vi "TCP Write Alive.vi"() -> ()   [LabVIEW 2011]
uses:
  <vilib>/Utility/tcp.llb/UDP Multicast Read-Only Open.vi
panel:
  in  "remote port or service name 2":u16=6341
  in  "address 2":string="localhost"
  in  "Name 2":string="MyName2>>"
  in  "OK":bool
  in  "MultiCast Address":string="234.5.6.7"
  out "Stopped":bool
  in  "MultiCast Port":u16=58432
  out "NaN/Path/Refnum? 2":bool
  out "concatenated string":string
  out "NaN/Path/Refnum?":bool
  in  "stop":bool
  in  "Name":string="MyName2>>"
  in  "Wait for Stop?":bool
  out "data out":string
  in  "remote port or service name":u16=6341
  in  "address":string="localhost"
  in  "timeout ms (25000)":i32
  out "connection ID out":refnum<k5>
  out "error out":errorcluster
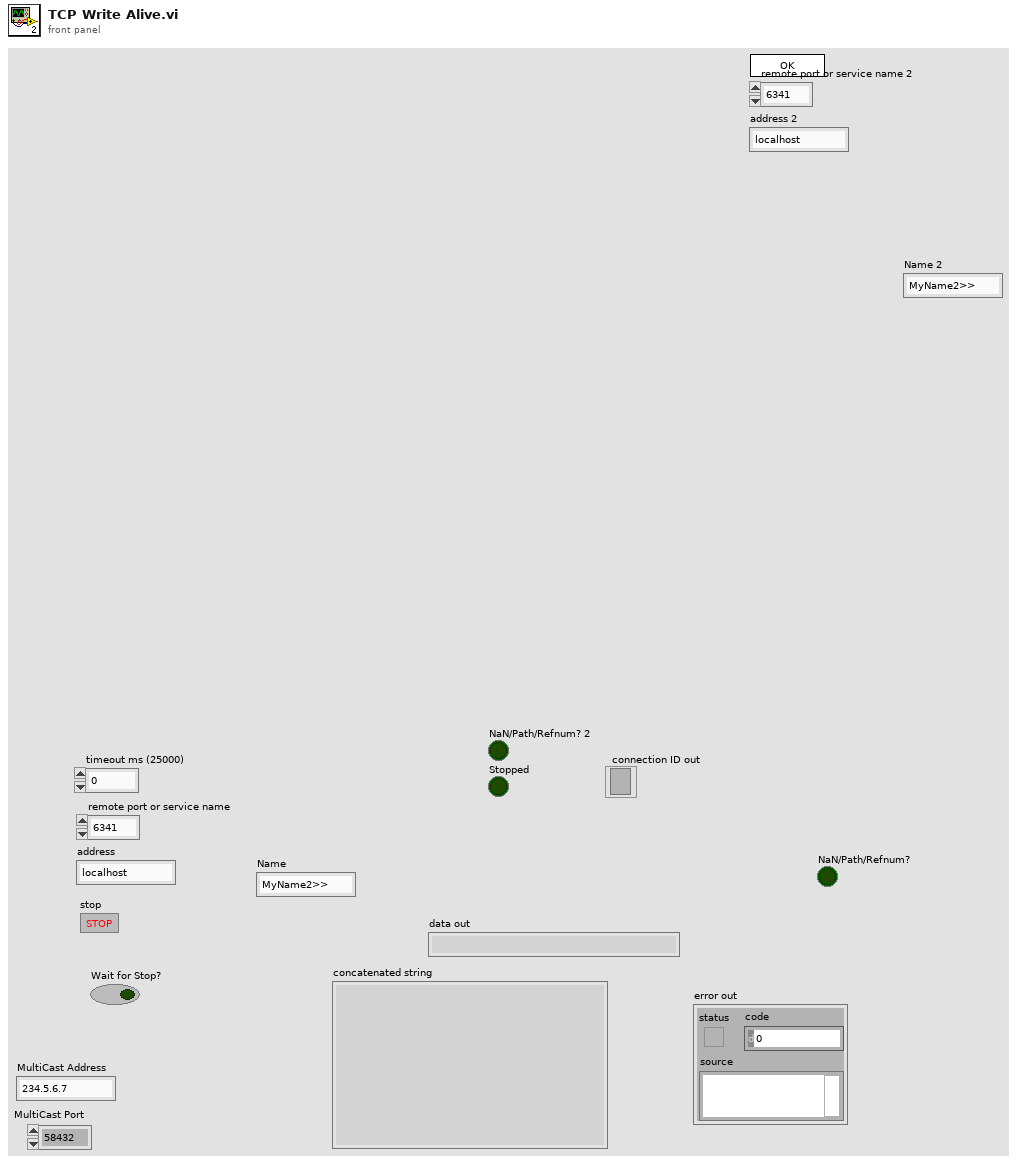
[diagram p1: front panel]
types:
  T1 = enum32{"invalid app kind", "Development System", "Run Time System", "Student Edition", "Embedded LabVIEW", "Evaluation", "Custom"}
  T2 = enum32{"Invalid", "Standard", "Closed", "Hidden", "Minimized", "Maximized"}
  T3 = cluster{"Core":cluster{"Current VI Reference":refnum<vi>, "Close Panel on Exit?":bool}, "Your Boolean data":bool, "Alive String":string, "connection ID":refnum<k5>, "Address":string, "remote port or service name 2":u16, "Stop String":string}
  T4 = cluster{"Current VI Reference":refnum<vi>, "Close Panel on Exit?":bool}
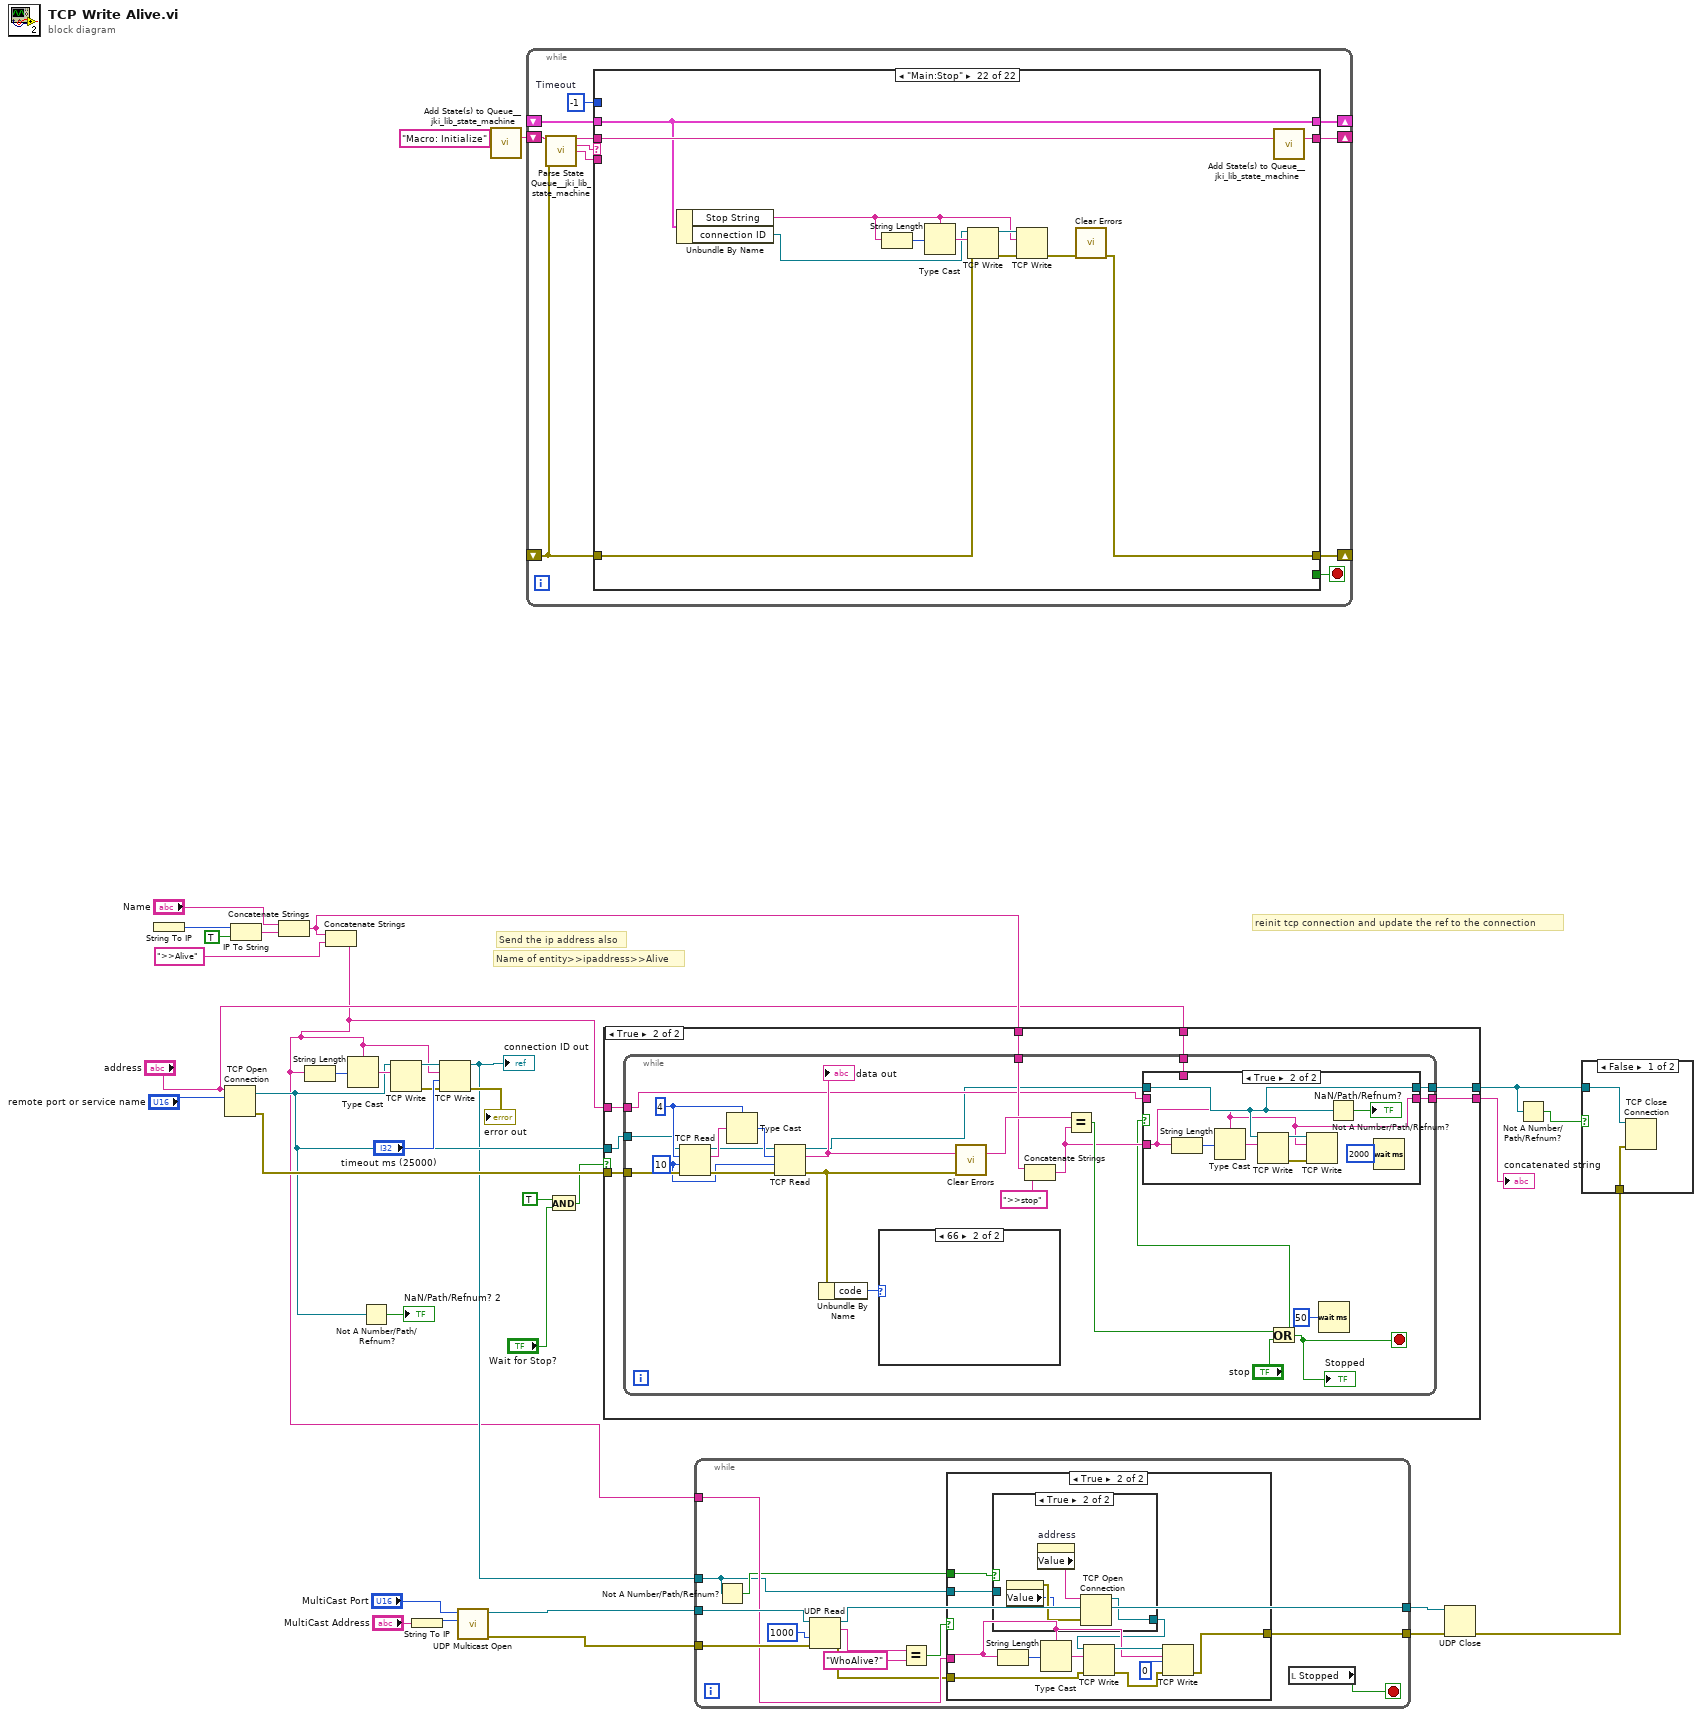
[diagram p0: block diagram]
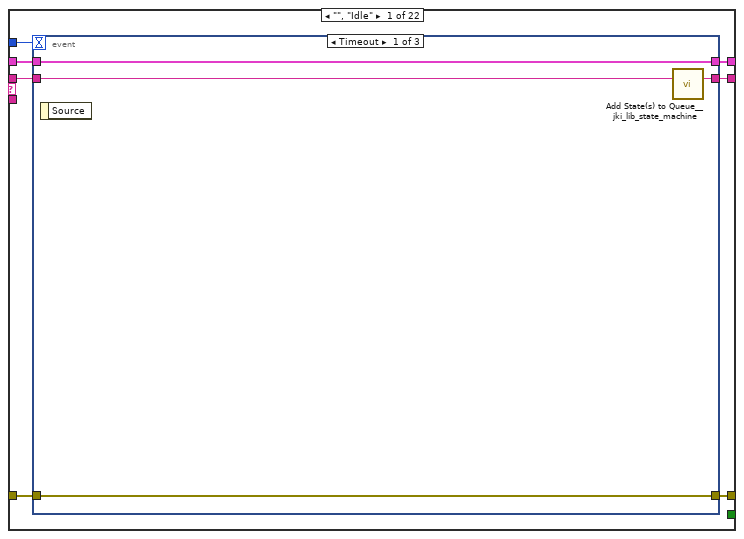
[diagram p2: hidden frame]
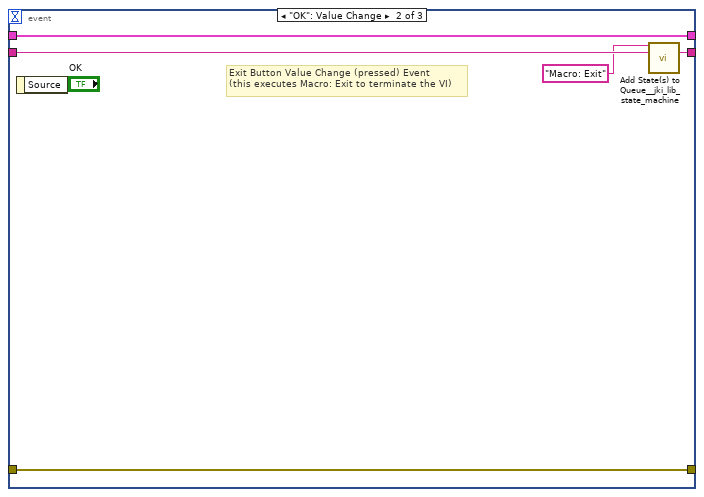
[diagram p3: hidden frame]
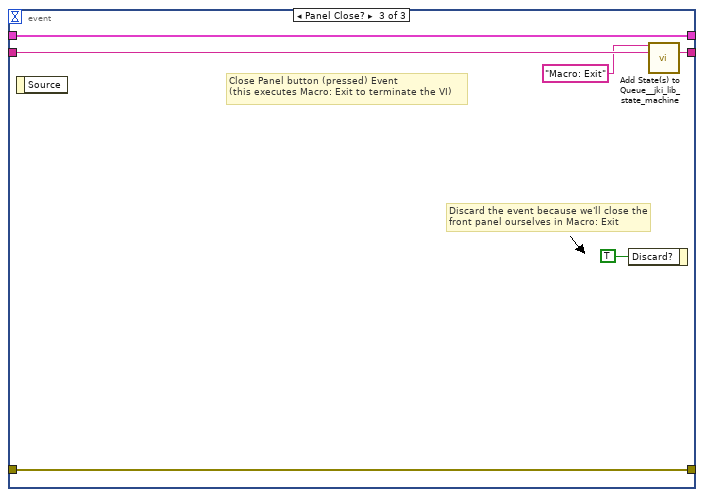
[diagram p4: hidden frame]
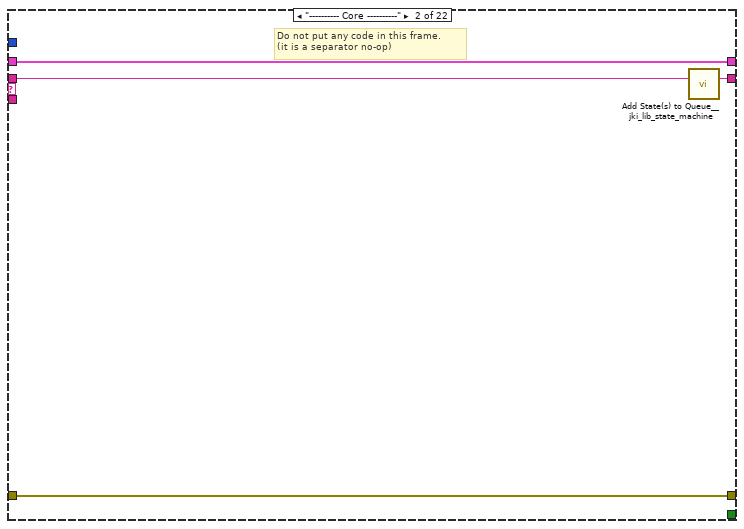
[diagram p5: hidden frame]
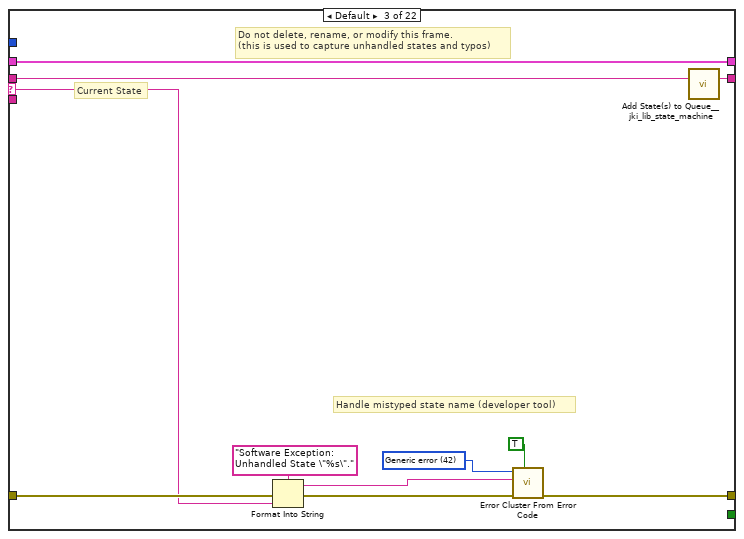
[diagram p6: hidden frame]
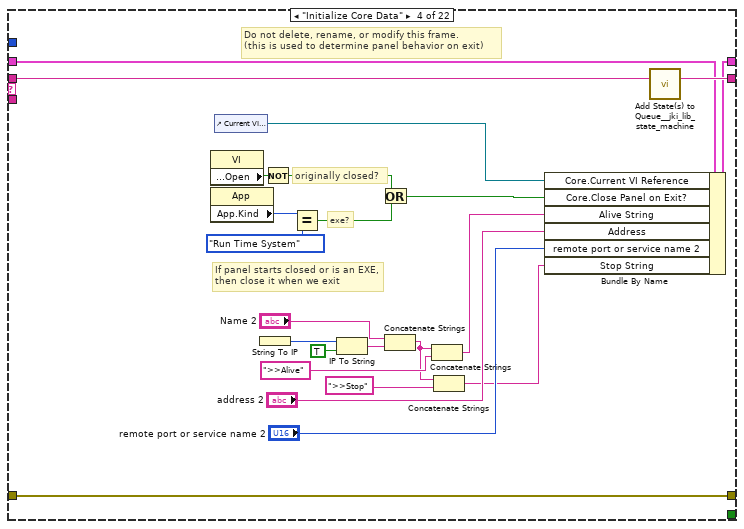
[diagram p7: hidden frame]
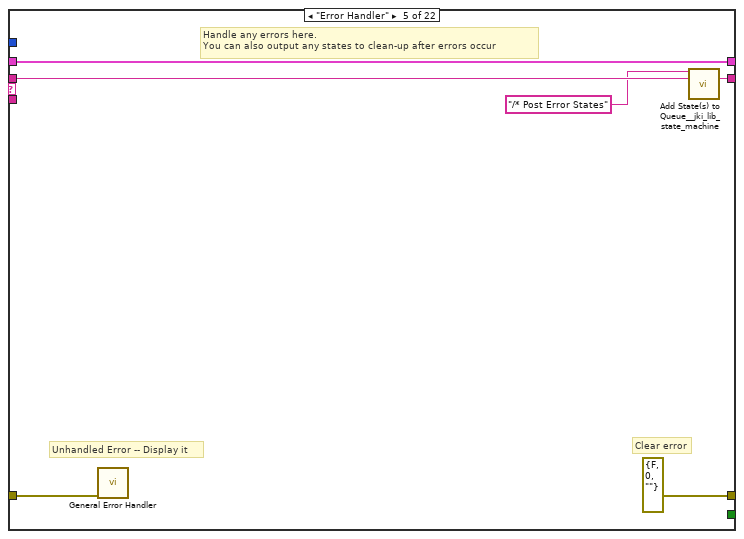
[diagram p8: hidden frame]
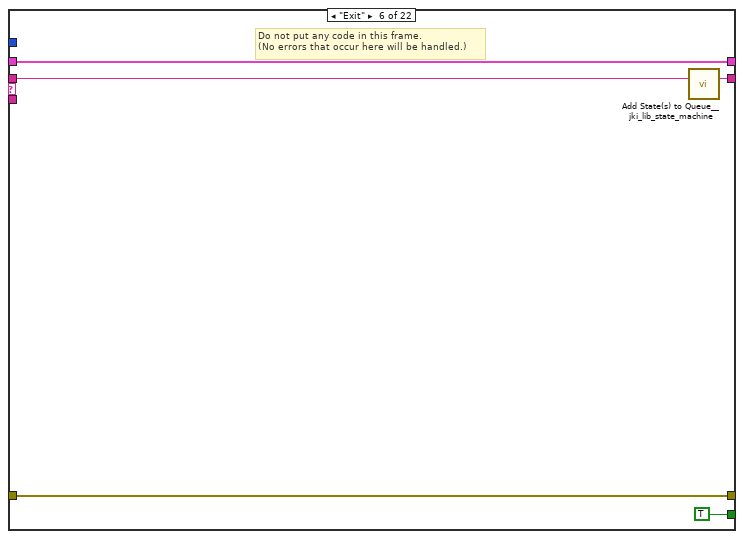
[diagram p9: hidden frame]
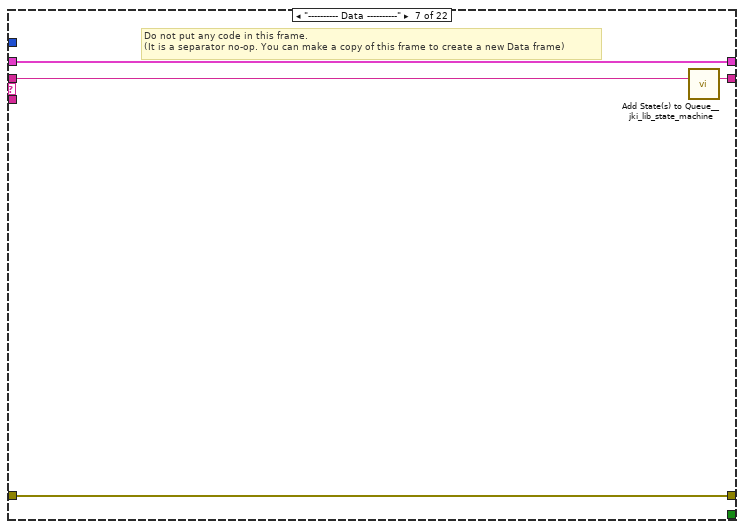
[diagram p10: hidden frame]
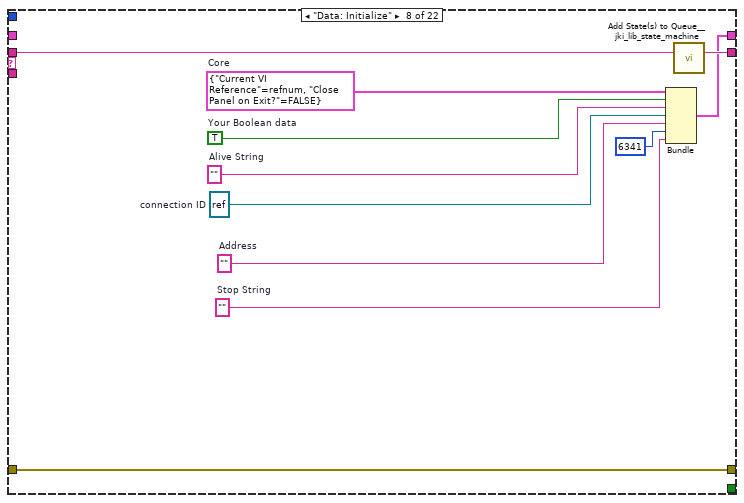
[diagram p11: hidden frame]
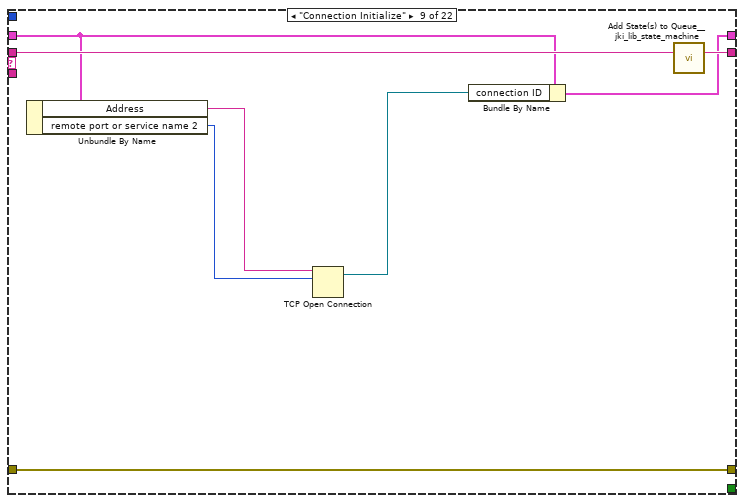
[diagram p12: hidden frame]
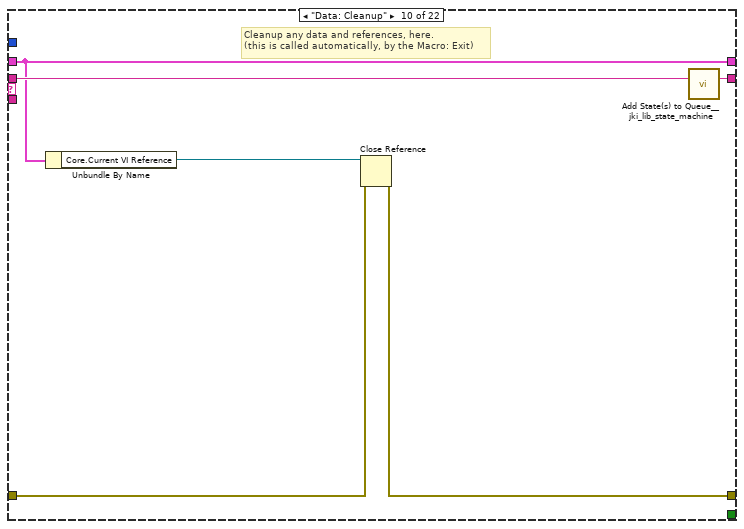
[diagram p13: hidden frame]
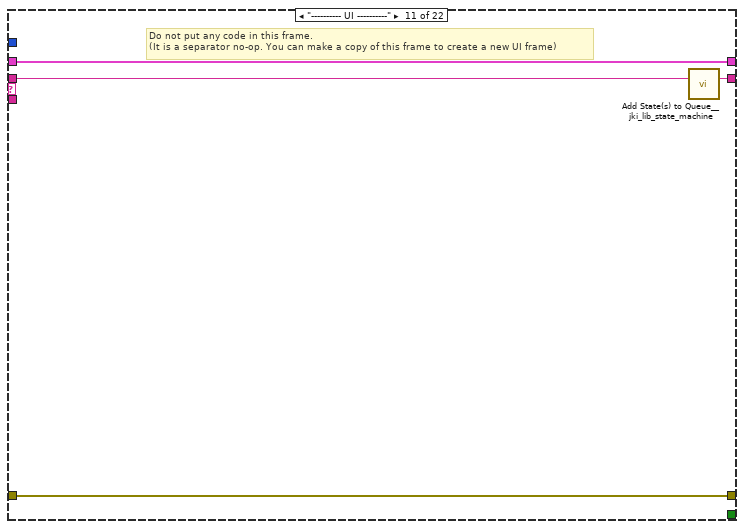
[diagram p14: hidden frame]
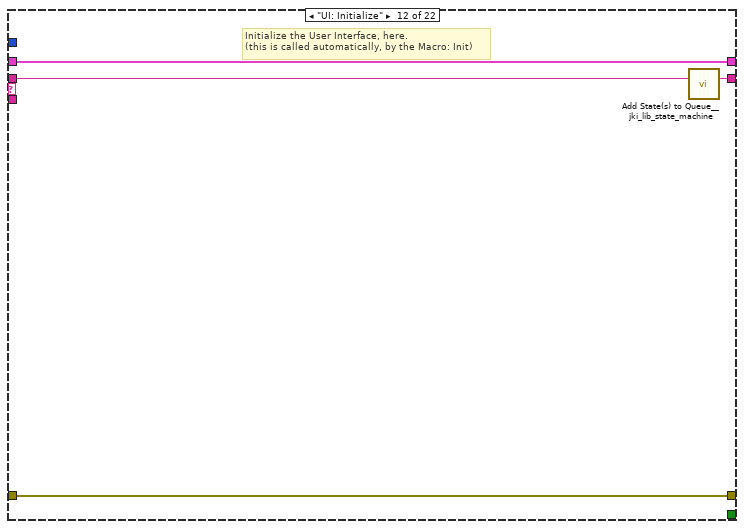
[diagram p15: hidden frame]
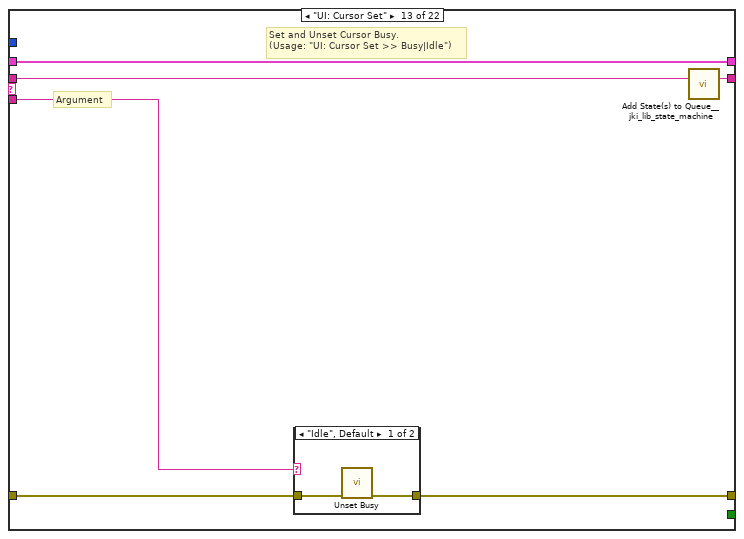
[diagram p16: hidden frame]
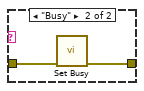
[diagram p17: hidden frame]
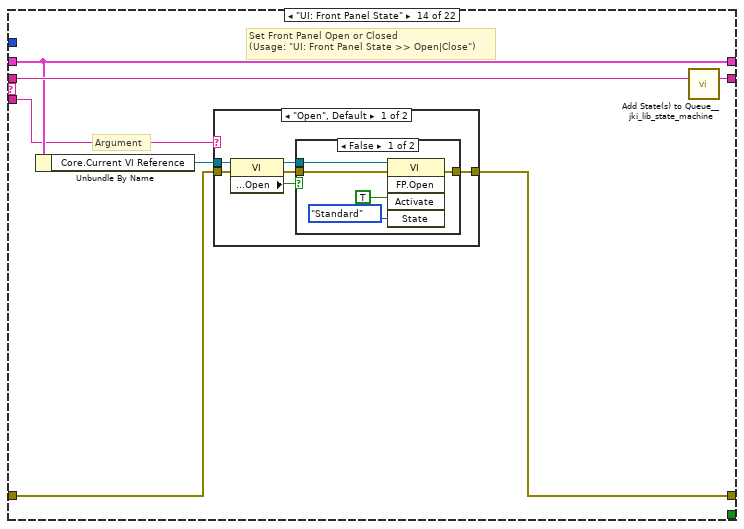
[diagram p18: hidden frame]
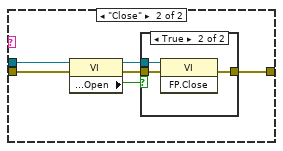
[diagram p20: hidden frame]
diagram:
  # "reinit tcp connection and update the ref to the connection"
  # "Send the ip address also"
  # "Name of entity>>ipaddress>>Alive"
  n1 = String To IP() -> (0:w24:u32)  [unwired: 1 in]
  n2 = TCP Open Connection(address="address", remote port or service name="remote port or service name") -> (connection ID=w15:refnum<k5>, error out=w29:errorcluster)  [unwired: 3 in]
  n3 = IP To String(1:TRUE ("dot notation? (F)"), 2:w24) -> (0:w22:string)
  n4 = Concatenate Strings("Name", w22) -> (w20:string)
  n5 = Concatenate Strings(w20, ">>Alive" ("string")) -> (w8:string)
  n6 = String Length(string=w8) -> (length=w31:i32)
  n7 = Type Cast(type=w8, x=w31) -> (*(type *) &x=w30:string)
  n8 = Not A Number/Path/Refnum?(number/path/refnum=w15) -> (NaN/Path/Refnum?=→"NaN/Path/Refnum? 2":bool)
  n9 = TCP Write(connection ID=w15, data in=w30) -> (connection ID out=w33:refnum<k5>, error out=w32:errorcluster)  [unwired: 2 in, 1 out]
  n10 = String To IP(1:"MultiCast Address") -> (0:w4:u32)
  n11 = TCP Write(connection ID=w33, data in=w8, error in (no error)=w32, 9:"timeout ms (25000)") -> (connection ID out=w9:refnum<k5>, error out=→"error out":errorcluster)  [unwired: 1 out]
  "connection ID out" <- w9
  n12 = call-poly <vilib>:"UDP Multicast Open.vi"("multicast addr"=w4, "port"="MultiCast Port") -> ("error out"=w11:errorcluster, "connection ID"=w10:refnum<k16>)  [unwired: 7 in, 1 out]
  n13 = call <vilib>:"Add State(s) to Queue__jki_lib_state_machine.vi"("State(s) in (\"\")"="Macro: Initialize") -> ("States Out"=w2:string)  [unwired: 14 in]
  n14 = while {
    shift-right: [w39] -> _
    shift-left: _ -> [w38]
    shift-right: [w42] -> _
    shift-left: _ -> [w36]
    shift-right: [w41] -> _
    shift-left: w2 -> [w43]
    stop <- w40 stop-if-true
    w37 = -1  # Timeout
    n15 = call <vilib>:"Parse State Queue__jki_lib_state_machine.vi"("State Queue"=w43, "Error In (no error)"=w36) -> ("Remaining States"=w45:string, "Current State"=w46:string, "Arguments"=w44:string)  [unwired: 11 in]
    n16 = case shown="\"Main:Stop\"" w46 {
      selector: w46 -> [_ _ w73 _ _ _ _ _ _ _ _ _ _ _ _ _ _ _ _ _ _ _]
      tunnel: w45 -> [w53 w72 w77 w106 w112 w117 w121 w132 w140 w146 w150 w154 w160 w171 w197 w202 w212 w216 w225 w242 w265 w277]
      tunnel: w44 -> [_ _ _ _ _ _ _ _ _ _ _ _ w155 w165 _ _ _ _ _ _ _ _]
      tunnel: w38 -> [w51 w69 w75 w97 w109 w115 w118 _ w135 w141 w147 w152 w158 w167 w194 w199 w209 w213 w219 w233 w259 w271]
      tunnel: [w50 w70 w79 w103 errorcluster {"status"=FALSE, "code"=0, "source"=""} ("error out") w114 w119 w129 w138 w142 w148 w151 w156 w168 w195 w200 w210 w214 w223 w227 w254 w266] -> w42
      tunnel: w36 -> [w49 w70 w78 w103 w108 w114 w119 w129 w138 w143 w148 w151 w157 w169 w195 w200 w210 w214 w223 w228 w256 w268]
      tunnel: [w52 w71 w76 w105 w111 w116 w120 w131 w139 w145 w149 w153 w159 w170 w196 w201 w211 w215 w224 w241 w264 w276] -> w41
      tunnel: [_ _ _ _ _ TRUE _ _ _ _ _ _ _ _ _ _ _ _ _ _ _ _] -> w40
      tunnel: [w48 w69 w75 w104 w109 w115 w118 w130 w137 w141 w147 w152 w158 w167 w194 w199 w209 w213 w218 w233 w259 w271] -> w39
      tunnel: w37 -> [w47 _ _ _ _ _ _ _ _ _ _ _ _ _ _ _ _ _ _ _ _ _]
      frame "", "Idle" {
        n17 = event shown="[0] Timeout" {
          selector: _ -> [_ _ _]
          dyn-events: _ -> [_ _ _]
          timeout: w47 -> [_ _ _]
          tunnel: w53 -> [w57 w62 w68]
          tunnel: [w56 w61 w67] -> w52
          tunnel: w51 -> [w54 w59 w65]
          tunnel: [w55 w60 w66] -> w50
          tunnel: w49 -> [w55 w60 w66]
          tunnel: [w54 w59 w65] -> w48
          event Timeout {
            n18 = event-data() -> ()  [unwired: 1 in, 1 out]
            n19 = call <vilib>:"Add State(s) to Queue__jki_lib_state_machine.vi"("State(s) in (\"\")"=w57) -> ("States Out"=w56:string)  [unwired: 14 in]
          }
          event "OK": Value Change {
            # "Exit Button Value Change (pressed) Event\n(this executes Macro: Exit to terminate the VI)"
            n20 = event-data() -> ()  [unwired: 1 in, 1 out]
            n21 = call <vilib>:"Add State(s) to Queue__jki_lib_state_machine.vi"("State(s) in Front (\"\")"="Macro: Exit", "State(s) in (\"\")"=w62) -> ("States Out"=w61:string)  [unwired: 13 in]
          }
          event Panel Close? {
            # "Discard the event because we'll close the front panel ourselves in Macro: Exit"
            # "Close Panel button (pressed) Event\n(this executes Macro: Exit to terminate the VI)"
            n22 = event-data() -> ()  [unwired: 1 in, 1 out]
            n23 = event-data("Discard?"=TRUE) -> ()  [unwired: 1 in, 1 out]
            n24 = call <vilib>:"Add State(s) to Queue__jki_lib_state_machine.vi"("State(s) in Front (\"\")"="Macro: Exit", "State(s) in (\"\")"=w68) -> ("States Out"=w67:string)  [unwired: 13 in]
          }
        }
      }
      frame "---------- Core ----------" {
        # "Do not put any code in this frame.\n(it is a separator no-op)"
        n25 = call <vilib>:"Add State(s) to Queue__jki_lib_state_machine.vi"("State(s) in (\"\")"=w72) -> ("States Out"=w71:string)  [unwired: 14 in]
      }
      frame Default {
        w82 = 42 items=["No error", "Argument error", "Memory is full", "Out of zone", "End of file", "File already open", "Generic file I/O error", "File not found", "File permission error", "Disk is full", "Duplicate path", "Too many files open", "System feature not enabled", "Resource file not found", "Cannot add resource", "Resource not found", "Image not found", "Image memory error", "Pen does not exist", "Config type invalid", "Config token not found", "Config parse error", "Config memory error", "Bad external code format", "Bad external code offset", "External code not present", "Null window", "Destroy window error", "Null menu", "Print aborted", "Bad print record", "Print driver error", "Windows error during printing", "Memory error during printing", "Print dialog error", "Generic print error", "Invalid device refnum", "Device not found", "Device parameter error", "Device unit error", "Cannot open device", "Device call aborted", "Generic error", "Cancelled by user", "Object ID too low", "Object ID too high", "Object not in heap", "Unknown heap", "Unknown object (invalid DefProc)", "Unknown object (DefProc not in table)", "Message out of range", "Invalid (null) method", "Unknown message", "Manager call not supported", "Bad address", "Network operation in progress", "Network operation timed out", "Connection is busy", "Network attribute not supported", "Network error", "Address in use", "System out of memory", "Connection aborted", "Connection refused", "Not connected", "Already connected", "Connection closed", "Initialization error (interapplication manager)", "Bad occurrence", "Wait on unbound occurrence handler", "Occurrence queue overflow", "Datalog type conflict", "Unused", "Unrecognized type (interapplication manager)", "Memory corrupt", "Failed to make temporary DLL", "Old CIN version", "Drag socket not found", "Failed to load drop-object", "Failed to register OLE object", "Failed to release OLE object", "Format specifier type mismatch", "Unknown format specifier", "Too few format specifiers", "Too many format specifiers", "Scan failed", "Newer CIN version", "Error converting to variant", "Runtime menu error", "Password tampered", "Variant attribute not found", "Incompatible variant data type", "Event data is not available", "Event Store is not present", "Occurrence is not found", "Event Queue is not created", "Event info is not available", "Refnum passed is NULL", "Error retrieving Class GUID", "Error retrieving CoClass GUID", "Error retrieving TypeLib GUID.", "Bad built application magic bytes.", "Specific driver is different from the specific driver associated with the Logical Name.", "There is no session opened to the class driver.", "Max Error", "MAX - Error with config objects", "MAX - Error loading configuration", "MAX - Group not supported"]
        # "Current State"
        # "Do not delete, rename, or modify this frame.\n(this is used to capture unhandled states and typos)"
        # "Handle mistyped state name (developer tool)"
        n26 = Format Into String(format string="Software Exception: Unhandled State \"%s\"." ("message"), error in=w78, w73) -> (resulting string=w81:string, error out=w80:errorcluster)  [unwired: 1 in]
        n27 = call <vilib>:"Error Cluster From Error Code.vi"("show call chain? (False)"=TRUE, "error in (no error)"=w80, "error message (\"\")"=w81, "error code (0)"=w82) -> ("error out"=w79:errorcluster)  [unwired: 5 in]
        n28 = call <vilib>:"Add State(s) to Queue__jki_lib_state_machine.vi"("State(s) in (\"\")"=w77) -> ("States Out"=w76:string)  [unwired: 14 in]
      }
      frame "Initialize Core Data" {
        # "Do not delete, rename, or modify this frame.\n(this is used to determine panel behavior on exit)"
        # "originally closed?"
        # "exe?"
        # "If panel starts closed or is an EXE, then close it when we exit"
        n29 = property class="VI"() -> ("Front Panel.Open"=w102:bool)  [unwired: 2 in, 2 out]
        n30 = property class="App"() -> ("App.Kind"=w101:T1)  [unwired: 2 in, 2 out]
        n31 = control-ref of="Current VI Reference"() -> (w95:refnum<vi>)
        n32 = String To IP() -> (0:w91:u32)  [unwired: 1 in]
        n33 = Not(x=w102) -> (.not. x?=w99:bool)
        n34 = Equal?(x=w101, y=T1."Run Time System" ("Application:Kind")) -> (x = y?=w98:bool)
        n35 = IP To String(1:TRUE ("dot notation? (F)"), 2:w91) -> (0:w93:string)
        n36 = Or(x=w99, y=w98) -> (x .or. y?=w96:bool)
        n37 = Concatenate Strings("Name 2", w93) -> (w86:string)
        n38 = Concatenate Strings(w86, ">>Alive" ("string")) -> (w87:string)
        n39 = Concatenate Strings(w86, ">>Stop" ("string")) -> (w84:string)
        n40 = Bundle By Name(cluster=w97, "Core.Current VI Reference"=w95, "Core.Close Panel on Exit?"=w96, "Alive String"=w87, "Address"="address 2", "remote port or service name 2"="remote port or service name 2", "Stop String"=w84) -> (w104:T3)
        n41 = call <vilib>:"Add State(s) to Queue__jki_lib_state_machine.vi"("State(s) in (\"\")"=w106) -> ("States Out"=w105:string)  [unwired: 14 in]
      }
      frame "Error Handler" {
        # "Unhandled Error -- Display it"
        # "Handle any errors here.\nYou can also output any states to clean-up after errors occur"
        # "Clear error"
        n42 = call <vilib>:"General Error Handler.vi"("error in (no error)"=w108) -> ()  [unwired: 10 in, 5 out]
        n43 = call <vilib>:"Add State(s) to Queue__jki_lib_state_machine.vi"("State(s) in Front (\"\")"="/* Post Error States", "State(s) in (\"\")"=w112) -> ("States Out"=w111:string)  [unwired: 13 in]
      }
      frame "Exit" {
        # "Do not put any code in this frame.\n(No errors that occur here will be handled.)"
        n44 = call <vilib>:"Add State(s) to Queue__jki_lib_state_machine.vi"("State(s) in (\"\")"=w117) -> ("States Out"=w116:string)  [unwired: 14 in]
      }
      frame "---------- Data ----------" {
        # "Do not put any code in this frame.\n(It is a separator no-op. You can make a copy of this frame to create a new Data frame)"
        n45 = call <vilib>:"Add State(s) to Queue__jki_lib_state_machine.vi"("State(s) in (\"\")"=w121) -> ("States Out"=w120:string)  [unwired: 14 in]
      }
      frame "Data: Initialize" {
        w122 = ""  # Stop String
        w124 = ""  # Address
        w125 = refnum<k5> refnum  # connection ID
        w126 = T4 {"Current VI Reference"=refnum, "Close Panel on Exit?"=FALSE}  # Core
        w128 = TRUE  # Your Boolean data
        w127 = ""  # Alive String
        n46 = Bundle("Core"=w126, "Your Boolean data"=w128, "Alive String"=w127, "connection ID"=w125, "Address"=w124, "remote port or service name 2"=u16 6341, "Stop String"=w122) -> (w130:T3)  [unwired: 1 in]
        n47 = call <vilib>:"Add State(s) to Queue__jki_lib_state_machine.vi"("State(s) in (\"\")"=w132) -> ("States Out"=w131:string)  [unwired: 14 in]
      }
      frame "Connection Initialize" {
        n48 = Unbundle By Name(w135) -> ("Address"=w134:string, "remote port or service name 2"=w133:u16)
        n49 = TCP Open Connection(address=w134, remote port or service name=w133) -> (connection ID=w136:refnum<k5>)  [unwired: 3 in, 1 out]
        n50 = Bundle By Name(cluster=w135, "connection ID"=w136) -> (w137:T3)
        n51 = call <vilib>:"Add State(s) to Queue__jki_lib_state_machine.vi"("State(s) in (\"\")"=w140) -> ("States Out"=w139:string)  [unwired: 14 in]
      }
      frame "Data: Cleanup" {
        # "Cleanup any data and references, here.\n(this is called automatically, by the Macro: Exit)"
        n52 = Unbundle By Name(w141) -> ("Core.Current VI Reference"=w144:refnum<vi>)
        n53 = Close Reference(reference=w144, error in (no error)=w143) -> (error out=w142:errorcluster)
        n54 = call <vilib>:"Add State(s) to Queue__jki_lib_state_machine.vi"("State(s) in (\"\")"=w146) -> ("States Out"=w145:string)  [unwired: 14 in]
      }
      frame "---------- UI ----------" {
        # "Do not put any code in this frame.\n(It is a separator no-op. You can make a copy of this frame to create a new UI frame)"
        n55 = call <vilib>:"Add State(s) to Queue__jki_lib_state_machine.vi"("State(s) in (\"\")"=w150) -> ("States Out"=w149:string)  [unwired: 14 in]
      }
      frame "UI: Initialize" {
        # "Initialize the User Interface, here.\n(this is called automatically, by the Macro: Init)"
        n56 = call <vilib>:"Add State(s) to Queue__jki_lib_state_machine.vi"("State(s) in (\"\")"=w154) -> ("States Out"=w153:string)  [unwired: 14 in]
      }
      frame "UI: Cursor Set" {
        # "Argument"
        # "Set and Unset Cursor Busy.\n(Usage: \"UI: Cursor Set >> Busy|Idle\")"
        n57 = case shown="\"Idle\", Default" w155 {
          tunnel: w157 -> [w162 w164]
          tunnel: [w161 w163] -> w156
          frame "Idle", Default {
            n58 = call <vilib>:"Unset Busy.vi"("error in (no error)"=w162) -> ("error out"=w161:errorcluster)  [unwired: 10 in]
          }
          frame "Busy" {
            n59 = call <vilib>:"Set Busy.vi"("error in (no error)"=w164) -> ("error out"=w163:errorcluster)  [unwired: 9 in, 1 out]
          }
        }
        n60 = call <vilib>:"Add State(s) to Queue__jki_lib_state_machine.vi"("State(s) in (\"\")"=w160) -> ("States Out"=w159:string)  [unwired: 14 in]
      }
      frame "UI: Front Panel State" {
        # "Argument"
        # "Set Front Panel Open or Closed\n(Usage: \"UI: Front Panel State >> Open|Close\")"
        n61 = Unbundle By Name(w167) -> ("Core.Current VI Reference"=w166:refnum<vi>)
        n62 = case shown="\"Open\", Default" w165 {
          tunnel: w169 -> [w175 w188]
          tunnel: [w177 w189] -> w168
          tunnel: w166 -> [w176 w186]
          frame "Open", Default {
            n63 = property class="VI"(reference=w176, error in=w175) -> (reference out=w173:refnum<vi>, error out=w174:errorcluster, "Front Panel.Open"=w172:bool)
            n64 = case shown="False" w172 {
              tunnel: [w180 w183] -> w177
              tunnel: w174 -> [w179 w183]
              tunnel: w173 -> [w178 _]
              frame False {
                n65 = invoke class="VI" method="FP.Open"(reference=w178, error in=w179, "Activate"=TRUE, "State"=T2."Standard") -> (error out=w180:errorcluster)  [unwired: 1 in, 4 out]
              }
              frame True {
              }
            }
          }
          frame "Close" {
            n66 = property class="VI"(reference=w186, error in=w188) -> (reference out=w185:refnum<vi>, error out=w187:errorcluster, "Front Panel.Open"=w184:bool)
            n67 = case shown="True" w184 {
              tunnel: [w190 w193] -> w189
              tunnel: w187 -> [w190 w192]
              tunnel: w185 -> [_ w191]
              frame False {
              }
              frame True {
                n68 = invoke class="VI" method="FP.Close"(reference=w191, error in=w192) -> (error out=w193:errorcluster)  [unwired: 1 in, 2 out]
              }
            }
          }
        }
        n69 = call <vilib>:"Add State(s) to Queue__jki_lib_state_machine.vi"("State(s) in (\"\")"=w171) -> ("States Out"=w170:string)  [unwired: 14 in]
      }
      frame "---------- Macro ----------" {
        # "Do not put any code in this frame.\n(It is a separator no-op. You can make a copy of this frame to create a new Macro frame)"
        n70 = call <vilib>:"Add State(s) to Queue__jki_lib_state_machine.vi"("State(s) in (\"\")"=w197) -> ("States Out"=w196:string)  [unwired: 14 in]
      }
      frame "Macro: Initialize" {
        w198 = "Data: Initialize\nInitialize Core Data\nConnection Initialize\nUI: Initialize\nUI: Front Panel State >> Open"  # Data: Initialize Initialize Core Data Connection Initialize UI: Initialize UI: Front Panel State >> Open
        # "Initialization Macro\n(This is called once, when the VI starts)"
        n71 = call <vilib>:"Add State(s) to Queue__jki_lib_state_machine.vi"("State(s) in Front (\"\")"=w198, "State(s) in (\"\")"=w202) -> ("States Out"=w201:string)  [unwired: 13 in]
      }
      frame "Macro: Exit" {
        # "Exit Macro\n(This is called once, when the VI exits)"
        n72 = Unbundle By Name(w209) -> ("Core.Close Panel on Exit?"=w208:bool)
        n73 = Select(t="UI: Front Panel State >> Close", s=w208, f="") -> (s? t:f=w205:string)
        n74 = call <vilib>:"Add State(s) to Queue__jki_lib_state_machine.vi"("State(s) in (\"\")"=w205, "State(s) at Back (\"\")"="Data: Cleanup\nExit") -> ("States Out"=w203:string)  [unwired: 13 in]
        n75 = call <vilib>:"Add State(s) to Queue__jki_lib_state_machine.vi"("State(s) in Front (\"\")"=w203, "State(s) in (\"\")"=w212) -> ("States Out"=w211:string)  [unwired: 13 in]
      }
      frame "---------- New Category ----------" {
        # "Template Separator\n(You can make a copy of, or modify, this frame)"
        n76 = call <vilib>:"Add State(s) to Queue__jki_lib_state_machine.vi"("State(s) in (\"\")"=w216) -> ("States Out"=w215:string)  [unwired: 14 in]
      }
      frame "Main: Reconnect" {
        # "Your code here.\n(You can make a copy of, or modify, this frame)"
        n77 = Unbundle By Name(w219) -> ("Address"=w221:string, "remote port or service name 2"=w220:u16)
        n78 = TCP Open Connection(address=w221, remote port or service name=w220) -> (connection ID=w222:refnum<k5>)  [unwired: 3 in, 1 out]
        n79 = Bundle By Name(cluster=w219, "connection ID"=w222) -> (w218:T3)
        n80 = call <vilib>:"Add State(s) to Queue__jki_lib_state_machine.vi"("State(s) in Front (\"\")"="Main: read" ("State(s) in Front (\"\")"), "State(s) in (\"\")"=w225) -> ("States Out"=w224:string)  [unwired: 13 in]
      }
      frame "Main: read" {
        w239 = 10 ("timeout ms (25000)")
        w235 = 4
        # "Your code here.\n(You can make a copy of, or modify, this frame)"
        n81 = Unbundle By Name(w233) -> ("Stop String"=w230:string, "connection ID"=w232:refnum<k5>)
        n82 = TCP Read(connection ID=w232, bytes to read=w235, error in (no error)=w228, 9:w239) -> (connection ID out=w237:refnum<k5>, data out=w234:string, error out=w238:errorcluster)  [unwired: 1 out]
        n83 = Type Cast(type=w235, x=w234) -> (*(type *) &x=w236:i32)
        n84 = TCP Read(connection ID=w237, bytes to read=w236, error in (no error)=w238, 9:w239) -> (data out=w231:string, error out=w229:errorcluster)  [unwired: 2 out]
        n85 = Unbundle By Name(w229) -> ("code"=w240:i32)
        n86 = case shown="0, Default" w240 {
          tunnel: w231 -> [w248 _]
          tunnel: w230 -> [w247 _]
          tunnel: w229 -> [w246 w252]
          tunnel: [w245 w251] -> w227
          tunnel: [w244 "Main: Reconnect" ("State(s) in Front (\"\")")] -> w226
          frame 0, Default {
            n87 = call <vilib>:"Clear Errors.vi"("error in (no error)"=w246) -> ("error out"=w245:errorcluster)  [unwired: 6 in]
            n88 = Equal?(x=w247, y=w248) -> (x = y?=w243:bool)
            n89 = case shown="True" w243 {
              tunnel: ["Main: read" ("State(s) in Front (\"\")") "Main:Stop" ("State(s) in Front (\"\")")] -> w244
              frame False {
              }
              frame True {
              }
            }
          }
          frame 66 {
            n90 = call <vilib>:"Clear Errors.vi"("error in (no error)"=w252) -> ("error out"=w251:errorcluster)  [unwired: 6 in]
          }
        }
        n91 = call <vilib>:"Add State(s) to Queue__jki_lib_state_machine.vi"("State(s) in Front (\"\")"=w226, "State(s) in (\"\")"=w242) -> ("States Out"=w241:string)  [unwired: 13 in]
      }
      frame "Main: Write Alive" {
        n92 = Unbundle By Name(w259) -> ("Alive String"=w258:string, "connection ID"=w257:refnum<k5>)
        n93 = String Length(string=w258) -> (length=w262:i32)
        n94 = Type Cast(type=w258, x=w262) -> (*(type *) &x=w263:string)
        n95 = TCP Write(connection ID=w257, data in=w263, error in (no error)=w256) -> (connection ID out=w260:refnum<k5>, error out=w261:errorcluster)  [unwired: 1 in, 1 out]
        n96 = TCP Write(connection ID=w260, data in=w258, error in (no error)=w261) -> (error out=w255:errorcluster)  [unwired: 1 in, 2 out]
        n97 = call <vilib>:"Clear Errors.vi"("error in (no error)"=w255) -> ("error out"=w254:errorcluster)  [unwired: 6 in]
        n98 = call <vilib>:"Add State(s) to Queue__jki_lib_state_machine.vi"("State(s) in (\"\")"=w265) -> ("States Out"=w264:string)  [unwired: 14 in]
      }
      frame "Main:Stop" {
        n99 = Unbundle By Name(w271) -> ("Stop String"=w270:string, "connection ID"=w269:refnum<k5>)
        n100 = String Length(string=w270) -> (length=w274:i32)
        n101 = Type Cast(type=w270, x=w274) -> (*(type *) &x=w275:string)
        n102 = TCP Write(connection ID=w269, data in=w275, error in (no error)=w268) -> (connection ID out=w272:refnum<k5>, error out=w273:errorcluster)  [unwired: 1 in, 1 out]
        n103 = TCP Write(connection ID=w272, data in=w270, error in (no error)=w273) -> (error out=w267:errorcluster)  [unwired: 1 in, 2 out]
        n104 = call <vilib>:"Clear Errors.vi"("error in (no error)"=w267) -> ("error out"=w266:errorcluster)  [unwired: 6 in]
        n105 = call <vilib>:"Add State(s) to Queue__jki_lib_state_machine.vi"("State(s) in (\"\")"=w277) -> ("States Out"=w276:string)  [unwired: 14 in]
      }
    }
  }
  n106 = And(x=TRUE, y="Wait for Stop?") -> (x .and. y?=w27:bool)
  n107 = case shown="True" w27 {
    tunnel: w15 -> [w279 w284]
    tunnel: w29 -> [_ w286]
    tunnel: w20 -> [_ w285]
    tunnel: "address" -> [_ w283]
    tunnel: [w279 w282] -> w16
    tunnel: w8 -> [w278 w281]
    tunnel: [w278 w280] -> w13
    frame False {
    }
    frame True {
      n108 = while {
        tunnel: w286 -> [w306]
        tunnel: w285 -> [w301]
        tunnel: w284 -> [w294]
        tunnel: w283 -> [w295]
        tunnel: [w293] -> w282
        tunnel: w281 -> [w292]
        tunnel: [w291] -> w280
        stop <- w290 stop-if-true
        w299 = 10 ("timeout ms (25000)")
        w308 = 4
        n109 = TCP Read(connection ID=w294, bytes to read=w308, error in (no error)=w306, 9:w299) -> (connection ID out=w305:refnum<k5>, data out=w309:string, error out=w304:errorcluster)  [unwired: 1 out]
        n110 = Type Cast(type=w308, x=w309) -> (*(type *) &x=w307:i32)
        n111 = TCP Read(connection ID=w305, bytes to read=w307, error in (no error)=w304, 9:w299) -> (connection ID out=w289:refnum<k5>, data out=w302:string, error out=w288:errorcluster)  [unwired: 1 out]
        "data out" <- w302
        n112 = Unbundle By Name(w288) -> ("code"=w287:i32)
        n113 = case shown="66" w287 {
          frame 0, Default {
          }
          frame 66 {
          }
        }
        n114 = call <vilib>:"Clear Errors.vi"("error in (no error)"=w288) -> ()  [unwired: 6 in, 1 out]
        n115 = Concatenate Strings(w301, ">>stop" ("y")) -> (w298:string)
        n116 = Equal?(x=w302, y=w298) -> (x = y?=w300:bool)
        n117 = Or(x=w300, y="stop") -> (x .or. y?=w290:bool)
        "Stopped" <- w290
        n118 = case shown="True" w290 {
          tunnel: w298 -> [_ w312]
          tunnel: w295 -> [_ _]
          tunnel: w289 -> [w311 w314]
          tunnel: [w311 w314] -> w293
          tunnel: w292 -> [w310 _]
          tunnel: [w310 w312] -> w291
          frame False {
          }
          frame True {
            n119 = String Length(string=w312) -> (length=w318:i32)
            n120 = Type Cast(type=w312, x=w318) -> (*(type *) &x=w319:string)
            n121 = TCP Write(connection ID=w314, data in=w319) -> (connection ID out=w317:refnum<k5>, error out=w316:errorcluster)  [unwired: 2 in, 1 out]
            n122 = TCP Write(connection ID=w317, data in=w312, error in (no error)=w316) -> ()  [unwired: 1 in, 3 out]
            n123 = Not A Number/Path/Refnum?(number/path/refnum=w314) -> (NaN/Path/Refnum?=→"NaN/Path/Refnum?":bool)
            n124 = Wait (ms)(milliseconds to wait=u32 2000) -> ()  [unwired: 1 out]
          }
        }
        n125 = Wait (ms)(milliseconds to wait=u32 50) -> ()  [unwired: 1 out]
      }
    }
  }
  "concatenated string" <- w13
  n126 = while {
    tunnel: w11 -> [w331]
    tunnel: w10 -> [w330]
    tunnel: w9 -> [w320]
    tunnel: w8 -> [w327]
    tunnel: [w326] -> w7
    tunnel: [w323] -> w6
    stop <- w325 stop-if-true
    n127 = Not A Number/Path/Refnum?(number/path/refnum=w320) -> (NaN/Path/Refnum?=w321:bool)
    n128 = UDP Read(connection ID=w330, timeout ms (25000)=1000, 8:w331) -> (data out=w329:string, error out=w324:errorcluster, 3:w326:refnum<k16>)  [unwired: 1 in, 2 out]
    n129 = Equal?(x=w329, y="WhoAlive?") -> (x = y?=w322:bool)
    n130 = case shown="True" w322 {
      tunnel: w327 -> [_ w340]
      tunnel: w324 -> [w333 w339]
      tunnel: [w333 w337] -> w323
      tunnel: w321 -> [_ w336]
      tunnel: w320 -> [_ w334]
      frame False {
      }
      frame True {
        n131 = case shown="True" w336 {
          tunnel: [w345 w346] -> w335
          tunnel: w334 -> [w345 _]
          frame False {
          }
          frame True {
            n132 = property on="remote port or service name" class="DigNum (strict)"() -> (error out=w348:errorcluster, "Value"=w347:u16)  [unwired: 2 in, 1 out]
            n133 = property on="address" class="Str"() -> ("Value"=w349:string)  [unwired: 2 in, 2 out]
            n134 = TCP Open Connection(address=w349, remote port or service name=w347, error in (no error)=w348) -> (connection ID=w346:refnum<k5>)  [unwired: 2 in, 1 out]
          }
        }
        n135 = String Length(string=w340) -> (length=w343:i32)
        n136 = Type Cast(type=w340, x=w343) -> (*(type *) &x=w344:string)
        n137 = TCP Write(connection ID=w335, data in=w344, error in (no error)=w339) -> (connection ID out=w342:refnum<k5>, error out=w338:errorcluster)  [unwired: 1 in, 1 out]
        n138 = TCP Write(connection ID=w342, data in=w340, error in (no error)=w338, 9:0 ("timeout ms (25000)")) -> (error out=w337:errorcluster)  [unwired: 2 out]
      }
    }
    n139 = local read "Stopped"() -> (w325:bool)
  }
  n140 = UDP Close(connection ID=w7, 8:w6) -> (error out=w5:errorcluster)  [unwired: 1 out]
  n141 = Not A Number/Path/Refnum?(number/path/refnum=w16) -> (NaN/Path/Refnum?=w17:bool)
  n142 = case shown="False" w17 {
    tunnel: w16 -> [w351 _]
    tunnel: w5 -> [w350 _]
    frame False {
      n143 = TCP Close Connection(connection ID=w351, error in (no error)=w350) -> ()  [unwired: 1 in, 2 out]
    }
    frame True {
    }
  }
